vi "Create.vi"(10 "Size":T1) -> (3 "World out":refnum<class "World.lvclass">)   [LabVIEW 2020, in "World.lvclass"]
uses:
  World.lvclass
  Particle/Position.ctl
  World.lvclass/World.ctl
  Particle.lvclass
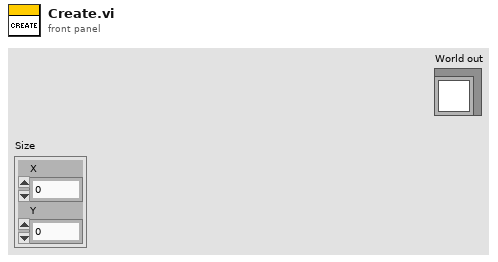
[diagram p1: front panel]
types:
  T1 = typedef "Particle.lvclass/Position.ctl" = cluster{"X":i32, "Y":i32}
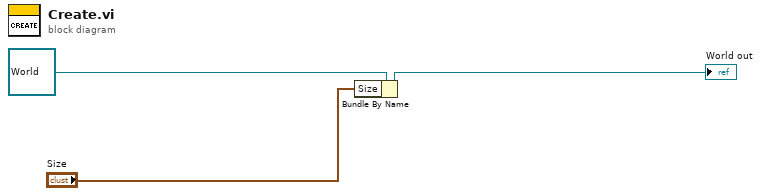
[diagram p0: block diagram]
diagram:
  n1 = Bundle By Name(cluster=refnum<class "World.lvclass"> refnum ("World in"), "Size"="Size") -> (→"World out":refnum<class "World.lvclass">)
